vi "Target Generate Gaussian Torque Setpoint Trajectory.vi"(11 "Torque Burst Parameters":T1) -> (0 "Phase Array (0-1)":dbl[](array[numeric]), 3 "Gaussian Torque Array (Nm)":dbl[](array[numeric]))   [LabVIEW 2018, in "COBRA Torque Setpoint Generators Library.lvlib"]
uses:
  COBRA Torque Setpoint Generators Library.lvlib
  Gaussian Torque Parameters.ctl
  <vilib>/Analysis/1siggen.llb/Ramp Pattern by Samples.vi
  <vilib>/Analysis/NI_AALBase.lvlib
panel:
  out "Torque vs Phase":cluster{"Ramp Pattern":dbl[], dbl[]}(graph)
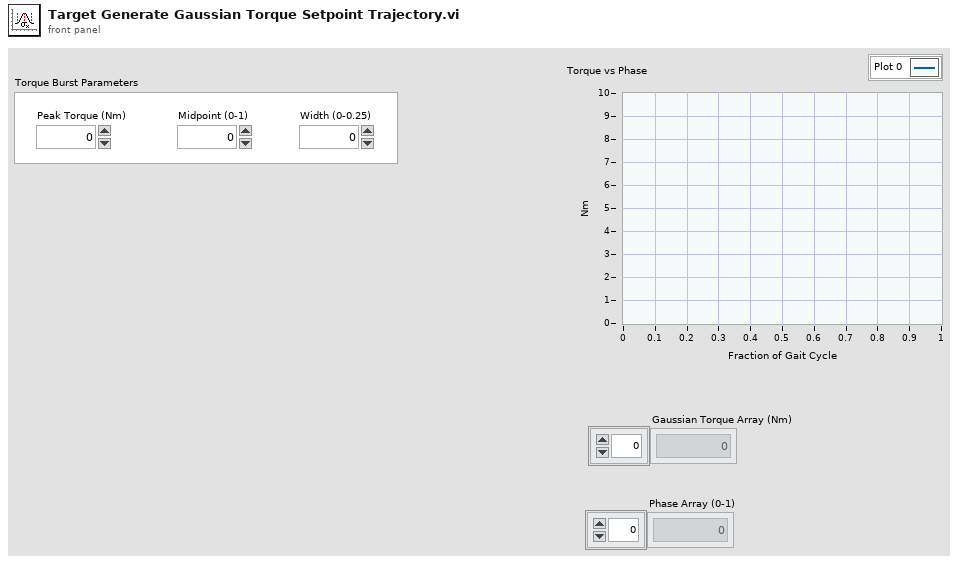
[diagram p1: front panel]
types:
  T1 = typedef "COBRA Torque Setpoint Generators Library.lvlib/Gaussian Torque Parameters.ctl" = cluster{"Peak Torque (Nm)":dbl, "Midpoint (0-1)":dbl, "Width (0-0.25)":dbl}
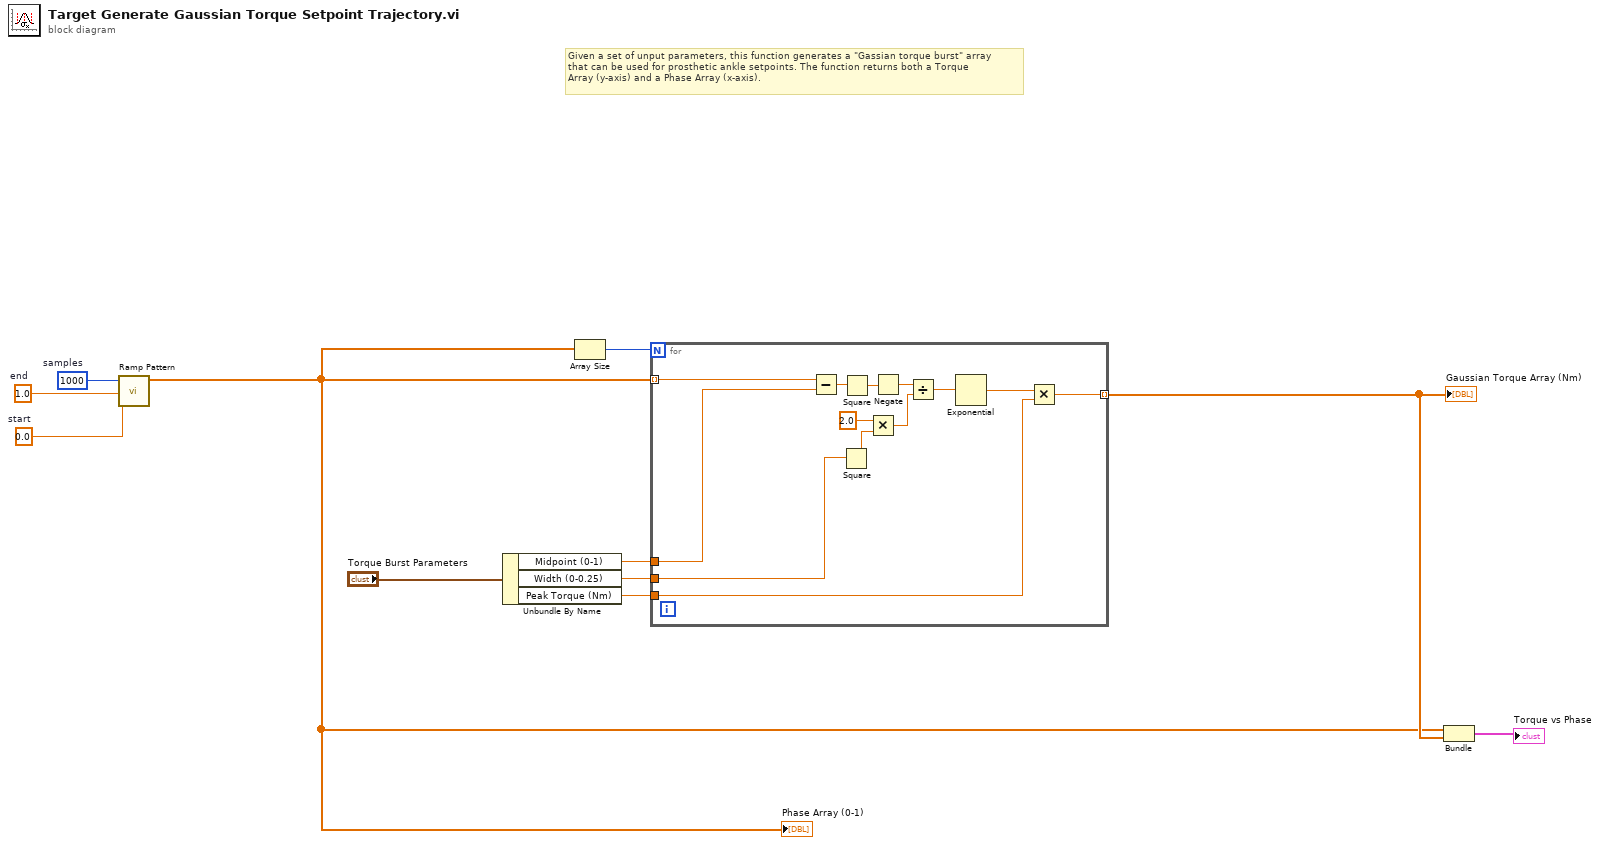
[diagram p0: block diagram]
diagram:
  w8 = 0.0  # start
  w9 = 1.0  # end
  w10 = 1000  # samples
  # "Given a set of unput parameters, this function generates a \"Gassian torque burst\" array\nthat can be used for prosthetic ankle setpoints. The function returns both a Torque\nArray (y-axis) and a Phase Array (x-axis)."
  n1 = call-poly <vilib>:"Ramp Pattern.vi"("start"=w8, "end"=w9, "samples"=w10) -> ("Ramp Pattern"=w1:dbl[])  [unwired: 7 in, 1 out]
  "Phase Array (0-1)" <- w1
  n2 = Unbundle By Name("Torque Burst Parameters") -> ("Midpoint (0-1)"=w4:dbl, "Width (0-0.25)"=w3:dbl, "Peak Torque (Nm)"=w2:dbl)
  n3 = Array Size(array=w1) -> (size(s)=w11:i32)
  n4 = for {
    N: w11 -> [_]
    tunnel: w1 -> [w16] mode=indexing
    tunnel: [w15] -> w6 mode=indexing
    tunnel: w4 -> [w14]
    tunnel: w3 -> [w13]
    tunnel: w2 -> [w12]
    n5 = Subtract(x=w16, y=w14) -> (x-y=w24:dbl)
    n6 = Square(x=w13) -> (x^2=w20:dbl)
    n7 = Square(x=w24) -> (x^2=w23:dbl)
    n8 = Multiply(x=2.0, y=w20) -> (x*y=w19:dbl)
    n9 = Negate(x=w23) -> (-x=w22:dbl)
    n10 = Divide(x=w22, y=w19) -> (x/y=w18:dbl)
    n11 = Exponential(1:w18) -> (0:w17:dbl)
    n12 = Multiply(x=w17, y=w12) -> (x*y=w15:dbl)
  }
  "Gaussian Torque Array (Nm)" <- w6
  n13 = Bundle("Ramp Pattern"=w1, w6) -> (→"Torque vs Phase":cluster{"Ramp Pattern":dbl[], dbl[]})  [unwired: 1 in]
